vi "Write State.vi"(8 "error in (no error)":errorcluster, 10 "State":refnum<class "State Pattern.lvclass">, 11 "Context in":refnum<class "Context.lvclass">) -> (0 "error out":errorcluster, 3 "Context out":refnum<class "Context.lvclass">)   [LabVIEW 2021, in "Context.lvlib" / "Context.lvclass"]
uses:
  Context.lvclass
  State Pattern/State Pattern/State Pattern.lvclass
  State/State.lvclass
  Context.lvclass/Context.ctl
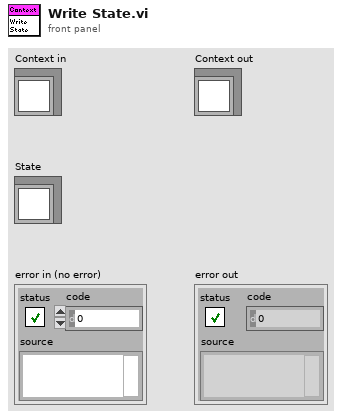
[diagram p1: front panel]
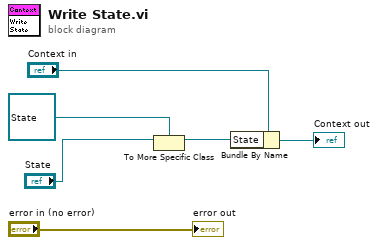
[diagram p0: block diagram]
diagram:
  n1 = To More Specific Class(target class=refnum<class "State.lvclass"> refnum ("Context Actor.lvlib:Context State.lvclass"), reference="State") -> (specific class reference=w2:refnum<class "State.lvclass">)  [unwired: 1 in, 1 out]
  n2 = Bundle By Name(cluster="Context in", "State"=w2) -> (→"Context out":refnum<class "Context.lvclass">)
  "error out" <- "error in (no error)"
